vi "PS Scan Control v0.80.vi"(2 "RampTo0?":bool=TRUE, 5 "Desired Field (T)":dbl format="%.2f", 7 "Slew Rate":dbl(slide)=10.0 scale=0.2..600.0 scale format="%.1f") -> (4 "Tesla":dbl(knob)=0.012045791994985122 caption="Current Field (T)" scale=0.0..20.0 scale format="%.1f")   [LabVIEW 2025]
doc: "Author: Scott Hannahs <sth@magnet.fsu.edu>\n\nThis software is licensed for use under the “MIT License\"\nCopyright (c) 2025 Scott Hannahs, sth@sth@magnet.sthnet.net\n\nPermission is hereby granted, free of charge, to any person obtaining a copy of this software and associated documentation files (the \"Software\"), to deal in the Software without restriction, including without limitation the rights to use, copy, modify, merge, publish, distribute, sublicense, and/or sell copies of the Software, and to permit persons to whom the Software is furnished to do so, subject to the following conditions: The above copyright notice and this permission notice shall be included in all copies or substantial portions of the Software.\n\nTHE SOFTWARE IS PROVIDED \"AS IS\", WITHOUT WARRANTY OF ANY KIND, EXPRESS OR IMPLIED, INCLUDING BUT NOT LIMITED TO THE WARRANTIES OF MERCHANTABILITY, FITNESS FOR A PARTICULAR PURPOSE AND NONINFRINGEMENT. IN NO EVENT SHALL THE AUTHORS OR COPYRIGHT HOLDERS BE LIABLE FOR ANY CLAIM, DAMAGES OR OTHER LIABILITY, WHETHER IN AN ACTION OF CONTRACT, TORT OR OTHERWISE, ARISING FROM, OUT OF OR IN CONNECTION WITH THE SOFTWARE OR THE USE OR OTHER DEALINGS IN THE SOFTWARE."
panel:
  in  "Current Tolerance":dbl=0.0049 min=0.0 max=30.0 format="%.1e"
  in  "stop":bool
  out "Cell":string
  in  "FRTZ":bool
  in  "Pause":bool
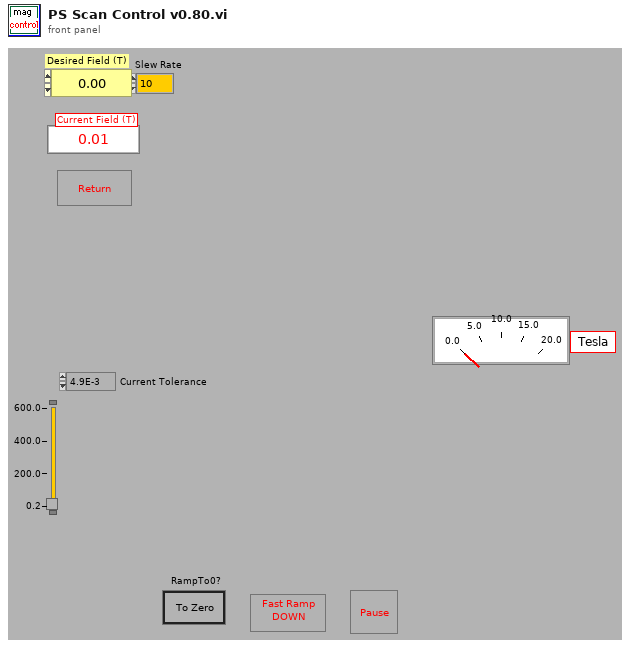
[diagram p1: front panel]
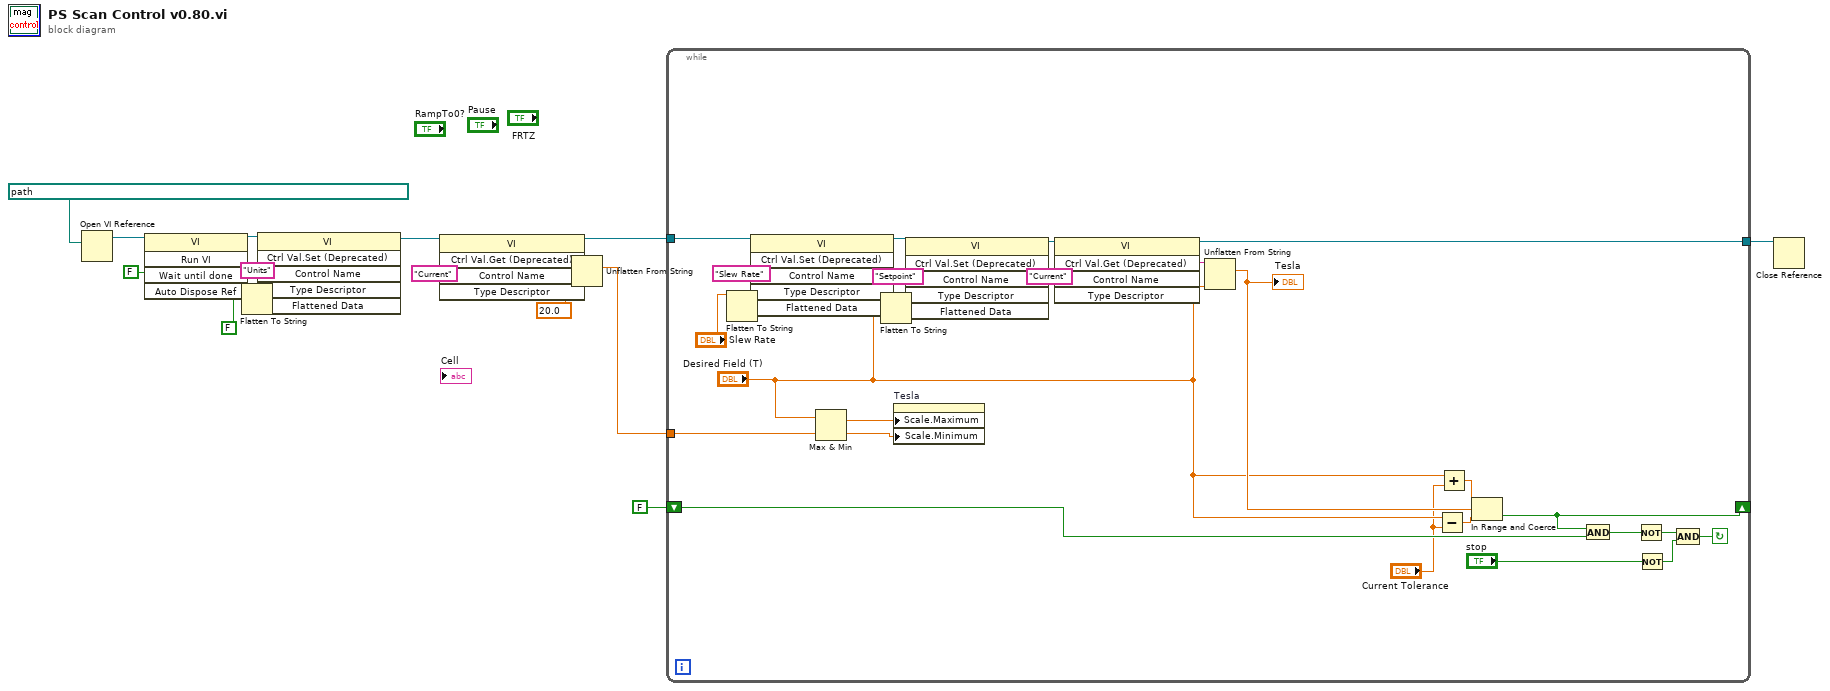
[diagram p0: block diagram]
diagram:
  n1 = Open VI Reference(vi path=path "/Optics2Mac/xwei Work/NML Data Acq/Serial Instruments/PS Ä/PS Control") -> (vi reference=w15:refnum<vi>)  [unwired: 5 in, 1 out]
  n2 = invoke class="VI" method="Run VI"(reference=w15, "Wait until done"=FALSE) -> (reference out=w8:refnum<vi>)  [unwired: 3 in, 4 out]
  n3 = Flatten To String(anything=FALSE ("Wait until done")) -> (data string=w12:string, type string=w11:i16[])  [unwired: 3 in, 1 out]
  n4 = invoke class="VI" method="Ctrl Val.Set (Deprecated)"(reference=w8, "Control Name"="Units", "Type Descriptor"=w11, "Flattened Data"=w12) -> (reference out=w5:refnum<vi>)  [unwired: 2 in, 5 out]
  n5 = invoke class="VI" method="Ctrl Val.Get (Deprecated)"(reference=w5, "Control Name"="Current") -> (reference out=w2:refnum<vi>, "Get Control Value"=w6:string)  [unwired: 3 in, 3 out]
  n6 = Unflatten From String(type=20.0 ("Desired Field (T)"), binary string=w6) -> (value=w3:dbl)  [unwired: 3 in, 2 out]
  n7 = while {
    tunnel: [w19] -> w1
    tunnel: w2 -> [w20]
    shift-left: FALSE -> [w34]
    shift-right: [w35] -> _
    tunnel: w3 -> [w37]
    stop <- w39 continue-if-true
    n8 = Flatten To String(anything="Slew Rate") -> (data string=w27:string, type string=w28:i16[])  [unwired: 3 in, 1 out]
    n9 = invoke class="VI" method="Ctrl Val.Set (Deprecated)"(reference=w20, "Control Name"="Slew Rate", "Type Descriptor"=w28, "Flattened Data"=w27) -> (reference out=w25:refnum<vi>)  [unwired: 2 in, 5 out]
    n10 = Max & Min(x="Desired Field (T)", y=w37) -> (max(x,y)=w38:dbl, min(x,y)=w36:dbl)
    n11 = Flatten To String(anything="Desired Field (T)") -> (data string=w30:string, type string=w31:i16[])  [unwired: 3 in, 1 out]
    n12 = property on="Tesla" class="Knob (strict)"("Scale.Maximum"=w38, "Scale.Minimum"=w36) -> ()  [unwired: 2 in, 2 out]
    n13 = invoke class="VI" method="Ctrl Val.Set (Deprecated)"(reference=w25, "Control Name"="Setpoint", "Type Descriptor"=w31, "Flattened Data"=w30) -> (reference out=w22:refnum<vi>)  [unwired: 2 in, 5 out]
    n14 = invoke class="VI" method="Ctrl Val.Get (Deprecated)"(reference=w22, "Control Name"="Current") -> (reference out=w19:refnum<vi>, "Get Control Value"=w23:string)  [unwired: 3 in, 3 out]
    n15 = Unflatten From String(type="Desired Field (T)", binary string=w23) -> (value=w21:dbl)  [unwired: 3 in, 2 out]
    "Tesla" <- w21
    n16 = Subtract(x="Desired Field (T)", y="Current Tolerance") -> (x-y=w42:dbl)
    n17 = Add(x="Desired Field (T)", y="Current Tolerance") -> (x+y=w43:dbl)
    n18 = In Range and Coerce(upper limit=w43, x=w21, lower limit=w42) -> (In Range?=w35:bool)  [unwired: 1 out]
    n19 = And(x=w35, y=w34) -> (x .and. y?=w33:bool)
    n20 = Not(x=w33) -> (.not. x?=w41:bool)
    n21 = Not(x="stop") -> (.not. x?=w40:bool)
    n22 = Compound Arithmetic op=AND(w41, w40) -> (w39:bool)
  }
  n23 = Close Reference(reference=w1) -> ()  [unwired: 1 in, 1 out]
